vi "E_hysteresis.vi"(4 "Low Comparitor":dbl, 5 "High Comparitor":dbl, 6 "Numeric":dbl, 7 "Previous State":bool) -> (2 "Output State":bool)   [LabVIEW 2013]
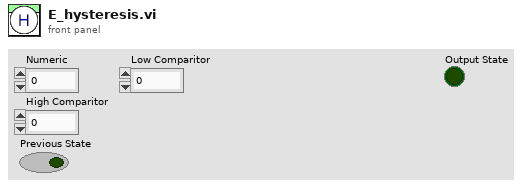
[diagram p1: front panel]
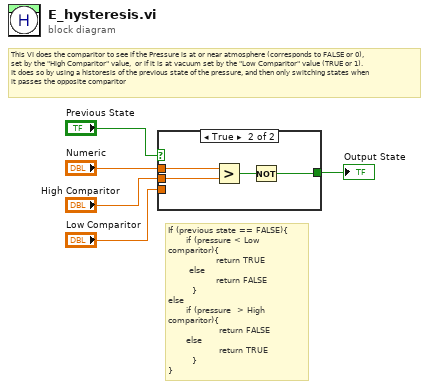
[diagram p0: block diagram]
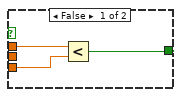
[diagram p2: hidden frame]
diagram:
  # "If (previous state == FALSE){\n      if (pressure < Low comparitor){ \n                return TRUE\n       else\n                return FALSE\n        }\nelse\n      if (pressure  > High comparitor){ \n                 return FALSE\n      else\n                 return TRUE\n        }\n}"
  # "This VI does the comparitor to see if the Pressure is at or near atmosphere (corresponds to FALSE or 0), \nset by the \"High Comparitor\" value,  or if it is at vacuum set by the \"Low Comparitor\" value (TRUE or 1). \nIt does so by using a historesis of the previous state of the pressure, and then only switching states when \nit passes the opposite comparitor"
  n1 = case shown="True" "Previous State" {
    tunnel: "Numeric" -> [w8 w12]
    tunnel: [w6 w10] -> w1
    tunnel: "High Comparitor" -> [_ w9]
    tunnel: "Low Comparitor" -> [w7 _]
    frame False {
      n2 = Less?(x=w8, y=w7) -> (x < y?=w6:bool)
    }
    frame True {
      n3 = Greater?(x=w12, y=w9) -> (0:w11:bool)
      n4 = Not(x=w11) -> (.not. x?=w10:bool)
    }
  }
  "Output State" <- w1
